vi "Check and compute displacements.vi"(8 "error in (no error)":errorcluster, 11 "Cascade in":refnum<class "Cascade.lvclass">) -> (0 "error out":errorcluster, 1 "fine?":bool, 2 "translation out":dbl[unit], 3 "Cascade out":refnum<class "Cascade.lvclass">)   [LabVIEW 2012, in "Cascade.lvclass"]
uses:
  Cascade.lvclass
  dependencies/ImageReg/Registration method.ctl
  Cascade.lvclass/Cascade.ctl
  <vilib>/Analysis/baseanly.llb/Mean (DBL).vi
  <vilib>/Analysis/NI_AALBase.lvlib
  <vilib>/gmath/NI_Gmath.lvlib
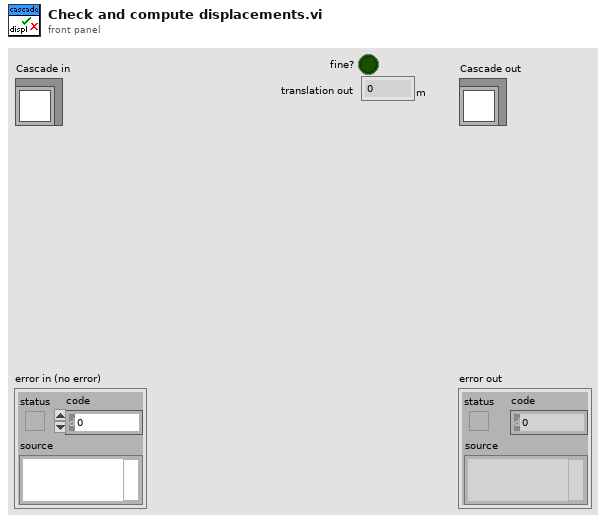
[diagram p1: front panel]
types:
  T1 = typedef "Registration method.ctl" = enum16{"Binarization", "Difference of Gaussians", "Edges Detection", "Gaussians and Binarization", "Edges and Gaussians", "Edges and Binarization", "All"}
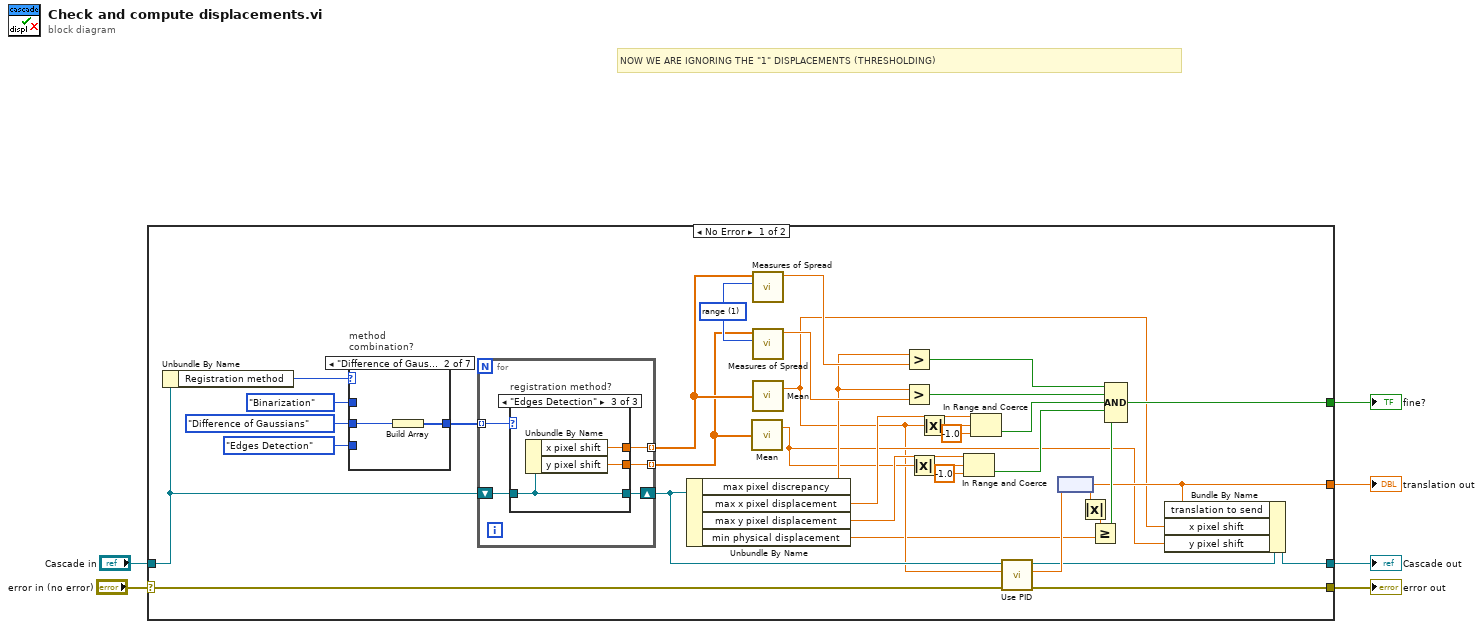
[diagram p0: block diagram]
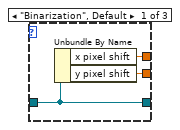
[diagram p2: hidden frame]
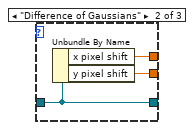
[diagram p3: hidden frame]
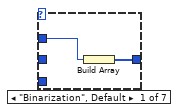
[diagram p4: hidden frame]
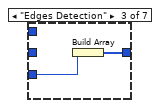
[diagram p5: hidden frame]
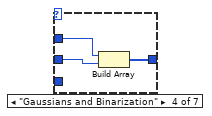
[diagram p6: hidden frame]
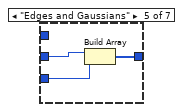
[diagram p7: hidden frame]
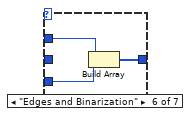
[diagram p8: hidden frame]
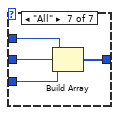
[diagram p9: hidden frame]
diagram:
  # "NOW WE ARE IGNORING THE \"1\" DISPLACEMENTS (THRESHOLDING)"
  n1 = case shown="No Error" "error in (no error)" {
    selector: "error in (no error)" -> [w16 w76]
    tunnel: [w14 w76] -> w5
    tunnel: [w12 w75] -> w3
    tunnel: "Cascade in" -> [w36 w75]
    tunnel: [w10 _] -> w2
    tunnel: [w11 _] -> w1
    frame No Error {
      w30 = 1 items=["standard deviation", "range", "mean absolute deviation", "interquartile range"] ("type")
      n2 = Unbundle By Name(w36) -> ("Registration method"=w38:T1)
      n3 = case "method\ncombination?" shown="\"Difference of Gaussians\"" w38 {
        tunnel: [w57 w59 w61 w64 w67 w70 w74] -> w37
        tunnel: Registration_method."Difference of Gaussians" ("Registration method") -> [_ w58 _ w62 w66 _ w71]
        tunnel: Registration_method."Binarization" ("Registration method") -> [w56 _ _ w63 _ w68 w73]
        tunnel: Registration_method."Edges Detection" ("Registration method") -> [_ _ w60 _ w65 w69 w72]
        frame "Binarization", Default {
          n4 = Build Array(w56) -> (w57:T1[])
        }
        frame "Difference of Gaussians" {
          n5 = Build Array(w58) -> (w59:T1[])
        }
        frame "Edges Detection" {
          n6 = Build Array(w60) -> (w61:T1[])
        }
        frame "Gaussians and Binarization" {
          n7 = Build Array(w63, w62) -> (w64:T1[])
        }
        frame "Edges and Gaussians" {
          n8 = Build Array(w66, w65) -> (w67:T1[])
        }
        frame "Edges and Binarization" {
          n9 = Build Array(w68, w69) -> (w70:T1[])
        }
        frame "All" {
          n10 = Build Array(w73, w71, w72) -> (w74:T1[])
        }
      }
      n11 = for {
        tunnel: w37 -> [w46] mode=indexing
        shift-right: [w44] -> w15
        shift-left: w36 -> [w45]
        tunnel: [w43] -> w22 mode=indexing
        tunnel: [w42] -> w21 mode=indexing
        n12 = case "registration method?" shown="\"Edges Detection\"" w46 {
          tunnel: w45 -> [w49 w52 w55]
          tunnel: [w49 w52 w55] -> w44
          tunnel: [w48 w51 w54] -> w43
          tunnel: [w47 w50 w53] -> w42
          frame "Binarization", Default {
            n13 = Unbundle By Name(w49) -> ("x pixel shift"=w48:dbl, "y pixel shift"=w47:dbl)
          }
          frame "Difference of Gaussians" {
            n14 = Unbundle By Name(w52) -> ("x pixel shift"=w51:dbl, "y pixel shift"=w50:dbl)
          }
          frame "Edges Detection" {
            n15 = Unbundle By Name(w55) -> ("x pixel shift"=w54:dbl, "y pixel shift"=w53:dbl)
          }
        }
      }
      n16 = Unbundle By Name(w15) -> ("max pixel discrepancy"=w20:dbl, "max x pixel displacement"=w19:dbl, "max y pixel displacement"=w18:dbl, "min physical displacement"=w7:dbl[unit])
      n17 = call-poly <vilib>:"Mean.vi"("X"=w21) -> ("mean"=w9:dbl)  [unwired: 1 out]
      n18 = call <vilib>:"Measures of Spread.vi"("type"=w30, "x array"=w22) -> ("spread value"=w31:dbl)  [unwired: 8 in, 1 out]
      n19 = call <vilib>:"Measures of Spread.vi"("type"=w30, "x array"=w21) -> ("spread value"=w32:dbl)  [unwired: 8 in, 1 out]
      n20 = call-poly <vilib>:"Mean.vi"("X"=w22) -> ("mean"=w8:dbl)  [unwired: 1 out]
      n21 = Greater?(x=w20, y=w31) -> (0:w29:bool)
      n22 = Greater?(x=w20, y=w32) -> (0:w33:bool)
      n23 = Absolute Value(x=w9) -> (abs(x)=w25:dbl)
      n24 = Absolute Value(x=w8) -> (abs(x)=w24:dbl)
      n25 = In Range and Coerce(upper limit=w18, x=w25, lower limit=-1.0) -> (In Range?=w34:bool)  [unwired: 1 out]
      n26 = In Range and Coerce(upper limit=w19, x=w24, lower limit=-1.0) -> (In Range?=w23:bool)  [unwired: 1 out]
      n27 = call-dynamic "Use PID.vi"("error in (no error)"=w16, "X pixel translation"=w8, "Cascade in"=w15) -> ("error out"=w14:errorcluster, "translation out"=w17:dbl, "Cascade out"=w13:refnum<class "Cascade.lvclass">)  [unwired: 6 in]
      n28 = node(w17) -> (w11:dbl[unit])
      n29 = Absolute Value(x=w11) -> (abs(x)=w28:dbl[unit])
      n30 = Greater Or Equal?(x=w28, y=w7) -> (x >= y?=w35:bool)
      n31 = Compound Arithmetic op=AND(w29, w33, w23, w34, w35) -> (w10:bool)
      n32 = Bundle By Name(cluster=w13, "translation to send"=w11, "x pixel shift"=w8, "y pixel shift"=w9) -> (w12:refnum<class "Cascade.lvclass">)
    }
    frame Error {
    }
  }
  "error out" <- w5
  "Cascade out" <- w3
  "fine?" <- w2
  "translation out" <- w1
